vi "CopyOneScan.vi"(8 "error in (no error)":errorcluster, 9 "block":u32=1, 10 "sample":u32=1, 11 "camera":u16=1) -> (0 "error out":errorcluster, 1 "Data Values Out 2":u16[](graph), 2 "Data Values Out 1":u16[](graph))   [LabVIEW 2015, in "ESLSCDLL.lvlib"]
uses:
  ESLSCDLL.lvlib
  Globals.vi
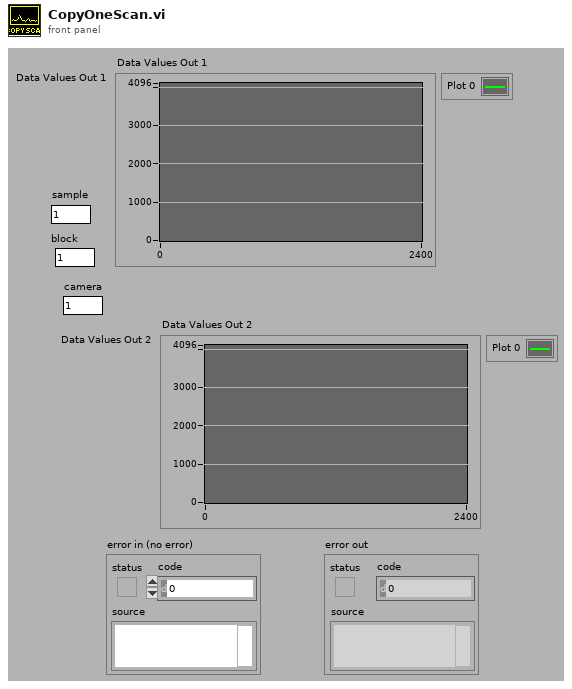
[diagram p1: front panel]
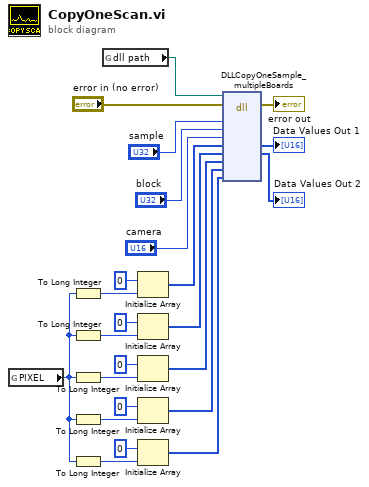
[diagram p0: block diagram]
diagram:
  n1 = global read "Globals.vi" "PIXEL"() -> (w5:u32)
  n2 = To Long Integer(number=w5) -> (32bit integer=w19:i32)
  n3 = To Long Integer(number=w5) -> (32bit integer=w16:i32)
  n4 = To Long Integer(number=w5) -> (32bit integer=w10:i32)
  n5 = To Long Integer(number=w5) -> (32bit integer=w8:i32)
  n6 = To Long Integer(number=w5) -> (32bit integer=w6:i32)
  n7 = global read "Globals.vi" "dll path"() -> (w1:path)
  n8 = Initialize Array(u16 0, w19) -> (w18:u16[])
  n9 = Initialize Array(u16 0, w16) -> (w12:u16[])
  n10 = Initialize Array(u16 0, w10) -> (w4:u16[])
  n11 = Initialize Array(u16 0, w8) -> (w3:u16[])
  n12 = Initialize Array(u16 0, w6) -> (w2:u16[])
  n13 = dll-call lib="C:/ENTW/PCIE/LV64/board.vis/ESLSCDLL.dll" fn="DLLCopyOneSample_multipleBoards" ("lwlscdll.dll:DLLReadFFLoop")(path in=w1, error in="error in (no error)", "sample"="sample", "block"="block", "camera"="camera", "pdest0"=w18, "pdest1"=w12, "pdest2"=w4, "pdest3"=w3, "pdest4"=w2) -> (error out=→"error out":errorcluster, "pdest0"=→"Data Values Out 1":u16[], "pdest1"=→"Data Values Out 2":u16[])  [unwired: 8 in, 1 out]
